vi "Lab03_2rng.vi"() -> ()   [LabVIEW 2022 SP3]
uses:
  <vilib>/numeric/Random Number (Range) DBL.vi
panel:
  out "XY Graph":cluster{dbl[], dbl[]}(graph)
  out "Numeric":dbl
  out "Sum of Difference Array":dbl[](array[numeric])
  out "Ran2":dbl[](array[numeric])
  out "Ran1":dbl[](array[numeric])
  out "Noisy Signal":dbl[][](graph)
  in  "# of Periods":dbl
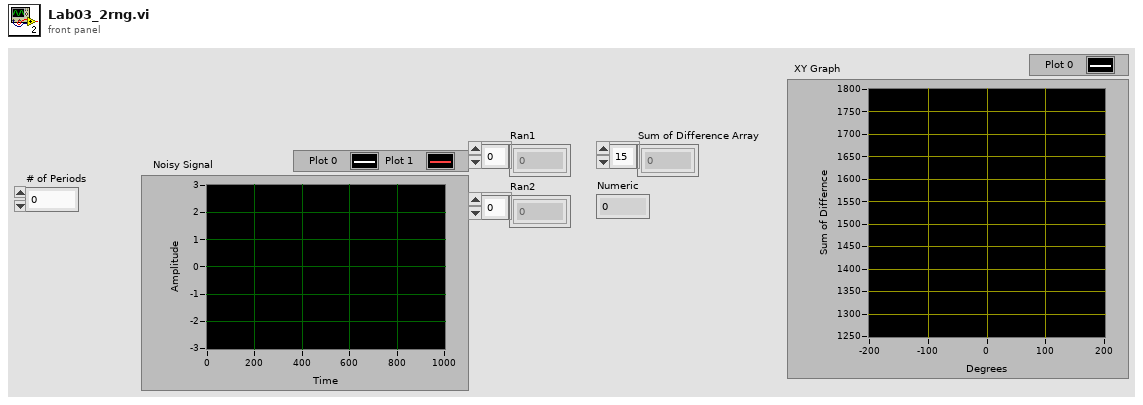
[diagram p1: front panel]
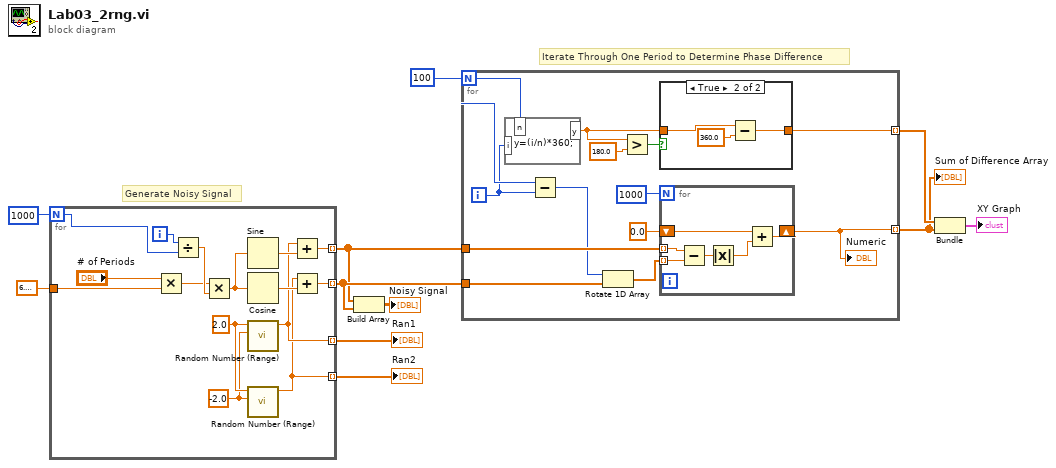
[diagram p0: block diagram]
diagram:
  # "Iterate Through One Period to Determine Phase Difference"
  # "Generate Noisy Signal"
  n1 = for {
    N: 1000 -> [w16]
    tunnel: [w18] -> w6 mode=indexing
    tunnel: [w15] -> w7 mode=indexing
    tunnel: [w14] -> w9 mode=indexing
    tunnel: [w13] -> w8 mode=indexing
    tunnel: 6.283185307179586 -> [w12]
    i -> [w17]
    w25 = -2.0 ("lower bound (0)")
    w26 = 2.0 ("upper bound (100)")
    n2 = Multiply(x="# of Periods", y=w12) -> (x*y=w22:dbl)
    n3 = Divide(x=w17, y=w16) -> (x/y=w23:dbl)
    n4 = Multiply(x=w22, y=w23) -> (x*y=w21:dbl)
    n5 = Sine(x=w21) -> (sin(x)=w19:dbl)
    n6 = Cosine(x=w21) -> (cos(x)=w20:dbl)
    n7 = call-poly <vilib>:"Random Number (Range).vi"("lower bound (0)"=w25, "upper bound (100)"=w26) -> ("number"=w14:dbl)  [unwired: 9 in]
    n8 = call-poly <vilib>:"Random Number (Range).vi"("lower bound (0)"=w25, "upper bound (100)"=w26) -> ("number"=w13:dbl)  [unwired: 9 in]
    n9 = Add(x=w14, y=w19) -> (x+y=w18:dbl)
    n10 = Add(x=w13, y=w20) -> (x+y=w15:dbl)
  }
  "Ran1" <- w9
  "Ran2" <- w8
  n11 = Build Array(w6, w7) -> (→"Noisy Signal":dbl[][])
  n12 = for {
    N: 100 -> [w29]
    tunnel: w7 -> [w36]
    tunnel: w6 -> [w39]
    tunnel: [w31] -> w3 mode=indexing
    tunnel: [w30] -> w2 mode=indexing
    i -> [w27]
    n13 = formula code="y=(i/n)*360;"("n"=w29, "i"=w27) -> ("y"=w32:dbl)
    n14 = Subtract(x=w29, y=w27) -> (x-y=w28:i32)
    n15 = Rotate 1D Array(1:w36, 2:w28) -> (0:w35:dbl[])
    n16 = Greater?(x=w32, y=180.0) -> (0:w34:bool)
    n17 = case shown="True" w34 {
      tunnel: w32 -> [w40 w43]
      tunnel: [w40 w41] -> w31
      frame False {
      }
      frame True {
        n18 = Subtract(x=w43, y=360.0) -> (x-y=w41:dbl)
      }
    }
    n19 = for {
      N: 1000 -> [_]
      tunnel: w35 -> [w44] mode=indexing
      tunnel: w39 -> [w49] mode=indexing
      shift-right: [w45] -> w30
      shift-left: 0.0 -> [w46]
      n20 = Subtract(x=w49, y=w44) -> (x-y=w48:dbl)
      n21 = Absolute Value(x=w48) -> (abs(x)=w47:dbl)
      n22 = Add(x=w46, y=w47) -> (x+y=w45:dbl)
    }
    "Numeric" <- w30
  }
  "Sum of Difference Array" <- w2
  n23 = Bundle(w3, w2) -> (→"XY Graph":cluster{dbl[], dbl[]})  [unwired: 1 in]
